vi "写入IMG设置.vi"(8 "error in (no error)":errorcluster caption="错误输入（无错误）", 10 "IMG设置":cluster{"IMG路径":path, "图片_高":dbl, "图片_宽":dbl}[](array[cluster]), 11 "EPUB输入":refnum<class "EPUB.lvclass">) -> (0 "error out":errorcluster caption="错误输出", 3 "EPUB输出":refnum<class "EPUB.lvclass">)   [LabVIEW 2016]
uses:
  EPUB.lvclass
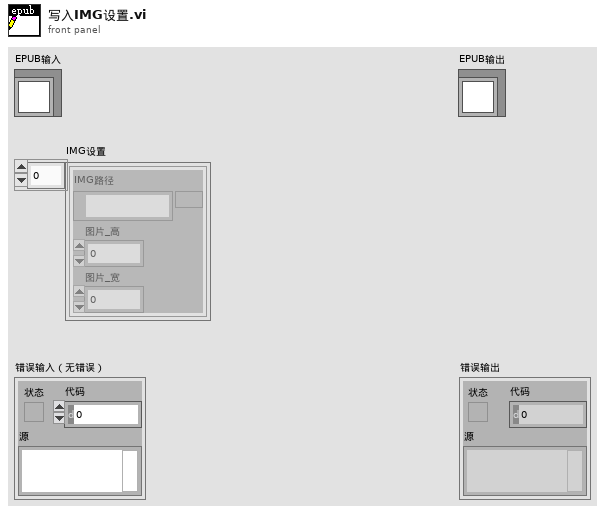
[diagram p1: front panel]
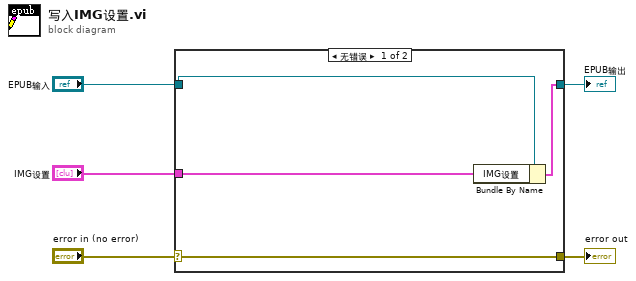
[diagram p0: block diagram]
diagram:
  n1 = case shown="无错误" "error in (no error)" {
    selector: "error in (no error)" -> [w9 w10]
    tunnel: [w9 w10] -> w4
    tunnel: [w7 w11] -> w2
    tunnel: "EPUB输入" -> [w8 w11]
    tunnel: "IMG设置" -> [w6 _]
    frame No Error {
      n2 = Bundle By Name(cluster=w8, "IMG设置"=w6) -> (w7:cluster{})
    }
    frame Error {
    }
  }
  "error out" <- w4
  "EPUB输出" <- w2
